vi "EV Rotator Shutdown.vi"(0 "Run Step Inputs":T1={"Data in"=[], "Results in"=[], "Seq Setup in"="", "Step name"="", "Hardware in"="", "Calibration in"="", "Step # in sequence"=0, "Display step?(f)"=TRUE, "Generate names only"=FALSE, "Waveforms in"=[], "Memory List Grouping info"=[]} {"Waveforms in"."Y dB ref" format="%.1f"; "Waveforms in"."Y axis" items=["dB", "Lin", "Pwr"]; "Waveforms in"."Y data" items=["dB", "Lin", "Pwr"]; "Waveforms in"."X data" items=["dB", "Lin", "Pwr"]; "Data in"."Z data" items=["dB", "Lin", "Pwr"]; "Data in"."X data" items=["dB", "Lin", "Pwr"]; "Data in"."Y data" items=["dB", "Lin", "Pwr"]; "Data in"."Z dB ref" format="%.1f"; "Data in"."Z axis" items=["Log", "Lin"]; "Data in"."X dB ref" format="%.1f"; "Data in"."X axis" items=["Log", "Lin"]; "Data in"."Y axis" items=["Log", "Lin"]; "Data in"."Y dB ref" format="%.1f"; "Data in"."Curve"."z" format="%.2f"; "Data in"."Curve"."y" format="%.2f"; "Data in"."Curve"."x" format="%.2f"; "Results in"."Unit type" items=["dB", "Lin", "Pwr"]; "Results in"."Margin" format="%.2f"}, 11 "error in (no error)":errorcluster) -> (6 "Data out":T2 {"Z data" items=["dB", "Lin", "Pwr"]; "X data" items=["dB", "Lin", "Pwr"]; "Y data" items=["dB", "Lin", "Pwr"]; "Z dB ref" format="%.1f"; "Z axis" items=["Log", "Lin"]; "X dB ref" format="%.1f"; "X axis" items=["Log", "Lin"]; "Y axis" items=["Log", "Lin"]; "Y dB ref" format="%.1f"; "Curve"."z" format="%.2f"; "Curve"."y" format="%.2f"; "Curve"."x" format="%.2f"}, 8 "Results out":T5 {"Unit type" items=["dB", "Lin", "Pwr"]; "Margin" format="%.2f"}, 10 "Waveforms out":T7 {"Y dB ref" format="%.1f"; "Y axis" items=["dB", "Lin", "Pwr"]; "Y data" items=["dB", "Lin", "Pwr"]; "X data" items=["dB", "Lin", "Pwr"]}, 15 "error out":errorcluster)   [LabVIEW 2018]
uses:
  custom and Sc run Seq Sub VIs (x64).llb/data array.ctl
  custom and Sc run Seq Sub VIs (x64).llb/data cluster.ctl
  custom and Sc run Seq Sub VIs (x64).llb/Axis Unit Type.ctl
  custom and Sc run Seq Sub VIs (x64).llb/result array.ctl
  custom and Sc run Seq Sub VIs (x64).llb/result cluster.ctl
  custom and Sc run Seq Sub VIs (x64).llb/waveform array.ctl
  custom and Sc run Seq Sub VIs (x64).llb/waveform cluster.ctl
  custom and Sc run Seq Sub VIs (x64).llb/Run Step Inputs.ctl
  custom and Sc run Seq Sub VIs (x64).llb/Memory List Grouping.ctl
  custom and Sc run Seq Sub VIs (x64).llb/Memory List Grouping - Item Type.ctl
  custom and Sc run Seq Sub VIs (x64).llb/window stack manager Functions.ctl
  C:/SoundCheck 19/System/Custom VIs/EV.Rotator.RotatorControl.dll
  EV.Rotator.RotatorControl.dll
panel:
  # "NOTE:  These controls and indicators must stay here, but you can Hide them if you wish.  These are wired as the standard input/output connector pane for step run VIs."
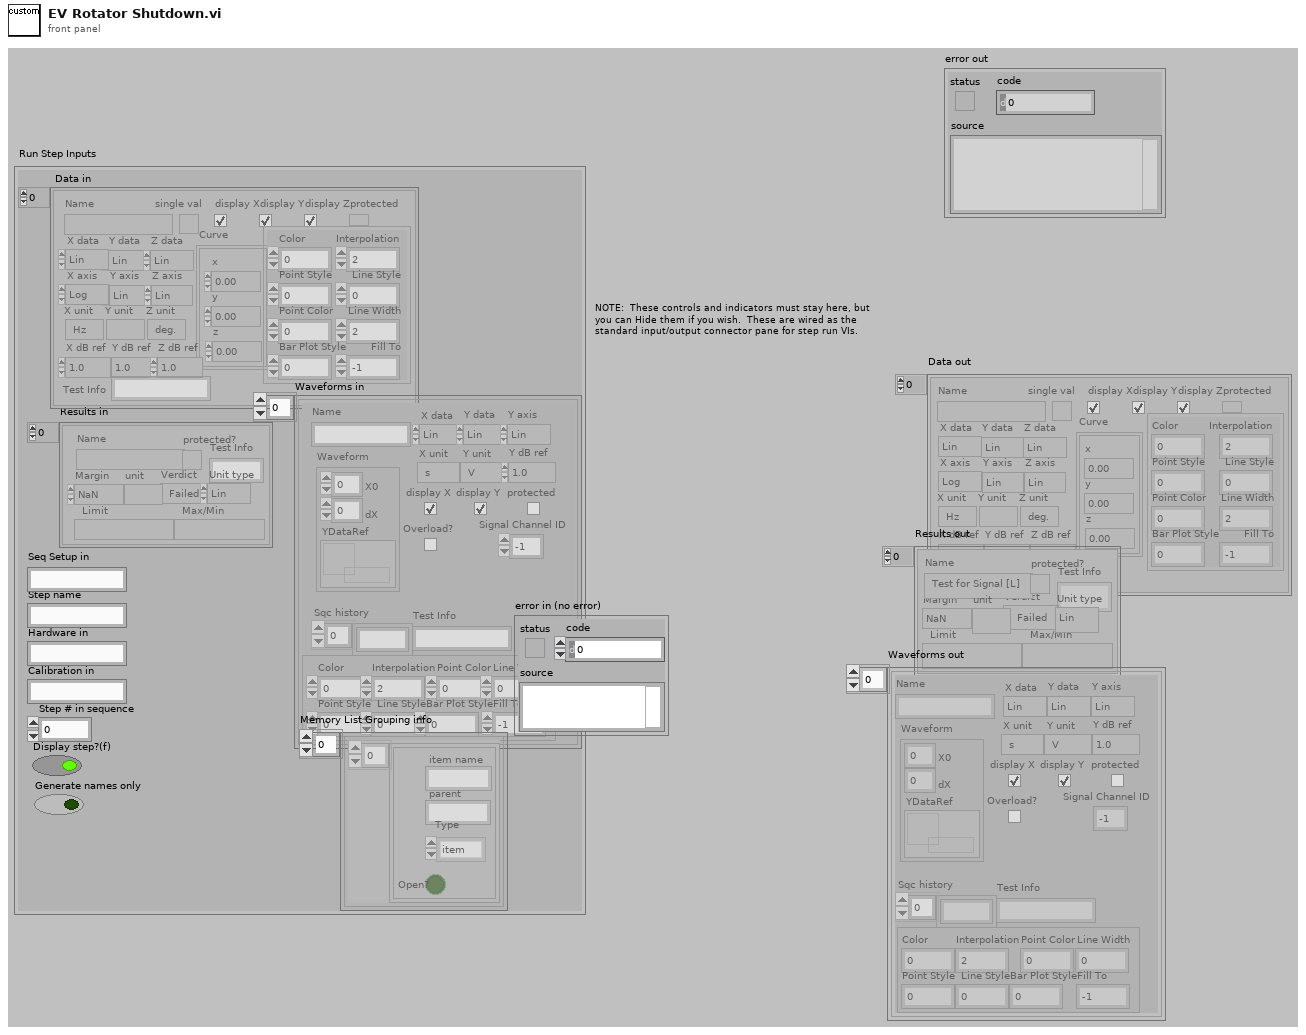
[diagram p1: front panel]
types:
  T1 = typedef "Run Step Inputs.ctl" = cluster{"Data in":T2, "Results in":T5, "Seq Setup in":string, "Step name":string, "Hardware in":string, "Calibration in":string, "Step # in sequence":i32, "Display step?(f)":bool, "Generate names only":bool, "Waveforms in":T7, "Memory List Grouping info":cluster{T9[]}[]}
  T2 = typedef "data array.ctl" = T3[]
  T3 = typedef "data cluster.ctl" = cluster{"Name":string, "Curve":cluster{"x":dbl, "y":dbl, "z":dbl}[], "X data":T4, "Y data":T4, "Z data":T4, "X axis":u16, "Y axis":u16, "Z axis":u16, "X unit":string, "Y unit":string, "Z unit":string, "X dB ref":dbl, "Y dB ref":dbl, "Z dB ref":dbl, "single val":bool, "protected":bool, "display X":bool, "display Y":bool, "display Z":bool, "Plot Settings":cluster{"Color":u32, "Interpolation":u8, "Point Style":u8, "Line Style":u8, "Point Color":u32, "Line Width":u8, "Bar Plot Style":u8, "Fill To":i16}, "Test Info":string}
  T4 = typedef "Axis Unit Type.ctl" = u16
  T5 = typedef "result array.ctl" = T6[]
  T6 = typedef "result cluster.ctl" = cluster{"Name":string, "Margin":dbl, "unit":string, "Verdict":bool, "Limit":string, "Max/Min":string, "protected?":bool, "Test Info":string, "Unit type":T4}
  T7 = typedef "waveform array.ctl" = T8[]
  T8 = typedef "waveform cluster.ctl" = cluster{"Name":string, "Waveform":cluster{"X0":dbl, "dX":dbl, "YDataRef":refnum<data-value>}, "X data":T4, "Y data":T4, "Y axis":T4, "X unit":string, "Y unit":string, "Y dB ref":dbl, "display Y":bool, "display X":bool, "Overload?":bool, "protected":bool, "Sqc history":string[], "Signal Channel ID":i32, "Plot Settings":cluster{"Color":u32, "Interpolation":u8, "Point Style":u8, "Line Style":u8, "Point Color":u32, "Line Width":u8, "Bar Plot Style":u8, "Fill To":i16}, "Test Info":string}
  T9 = typedef "Memory List Grouping.ctl" = cluster{"item name":string, "parent":string, "Open?":bool, "Type":T10}
  T10 = typedef "Memory List Grouping - Item Type.ctl" = enum16{"item", "custom group", "auto group", "protected group"}
  T11 = typedef "window stack manager Functions.ctl" = enum16{"Init", "add", "remove", "run", "clear", "vi stopped offset", "minimize all", "restore all", "autoadd", "Hourglass On", "Hourglass Off"}
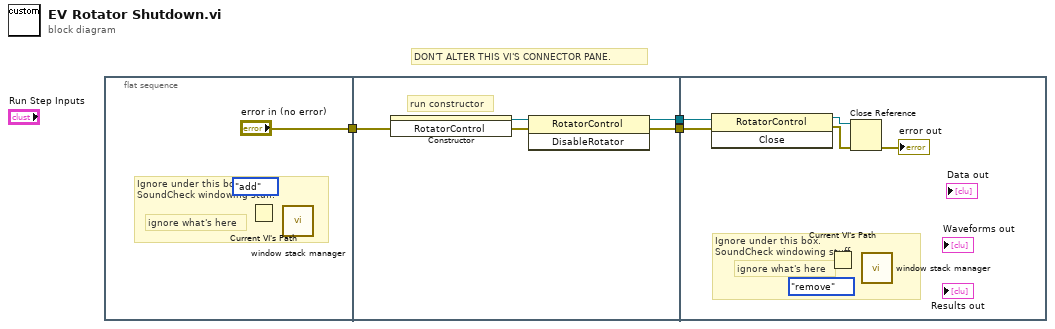
[diagram p0: block diagram]
diagram:
  # "DON'T ALTER THIS VI'S CONNECTOR PANE."
  n1 = flat-sequence {
    tunnel: ["error in (no error)"] -> w3
    tunnel: w3 -> [w9]
    tunnel: [w11] -> w2
    tunnel: [w10] -> w1
    tunnel: w2 -> [w13]
    tunnel: w1 -> [w12]
    frame #0 {
      # "Ignore under this box. \nSoundCheck windowing stuff."
      # "ignore what's here"
      n2 = Current VI's Path() -> (path=w6:path)
      n3 = call "window stack manager.vi"("VI path"=w6, "Function (run)"=window_stack_manager_Functions."add") -> ()  [unwired: 5 in, 5 out]
    }
    frame #1 {
      # "run constructor"
      n4 = constructor class="RotatorControl"(error in=w9) -> (reference out=w8:refnum<k24>, error out=w7:errorcluster)  [unwired: 2 in, 1 out]
      n5 = invoke class="RotatorControl" method="DisableRotator"(reference=w8, error in=w7) -> (reference out=w11:refnum<k24>, error out=w10:errorcluster)  [unwired: 1 in, 1 out]
    }
    frame #2 {
      # "Ignore under this box. \nSoundCheck windowing stuff."
      # "ignore what's here"
      n6 = invoke class="RotatorControl" method="Close"(reference=w13, error in=w12) -> (reference out=w14:refnum<k24>, error out=w15:errorcluster)  [unwired: 1 in, 1 out]
      n7 = Current VI's Path() -> (path=w18:path)
      n8 = Close Reference(reference=w14, error in (no error)=w15) -> (error out=→"error out":errorcluster)
      n9 = call "window stack manager.vi"("VI path"=w18, "Function (run)"=window_stack_manager_Functions."remove") -> ()  [unwired: 5 in, 5 out]
    }
  }
